vi "WriteFile.vi"() -> ()   [LabVIEW 2014]
panel:
  in  "name or relative path":string="FileIO.txt"
  in  "base path":path
  in  "text to file":string caption="text from file"
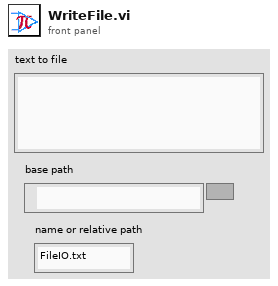
[diagram p1: front panel]
types:
  T1 = enum16{"open", "replace", "create", "open or create", "replace or create", "replace or create with confirmation"}
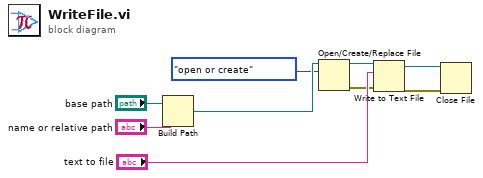
[diagram p0: block diagram]
diagram:
  n1 = Build Path(base path="base path", name or relative path="name or relative path") -> (appended path=w4:path)
  n2 = Open/Create/Replace File(file path (use dialog)=w4, operation (0:open)=T1."open or create") -> (refnum out=w2:refnum<file>, error out=w6:errorcluster)  [unwired: 4 in, 1 out]
  n3 = Write to Text File(file (use dialog)=w2, text="text to file", error in=w6) -> (refnum out=w1:refnum<file>, error out=w5:errorcluster)  [unwired: 1 in, 1 out]
  n4 = Close File(refnum=w1, error in=w5) -> ()  [unwired: 2 out]
